vi "Read Decimated Traces.vi"(8 "Error In":errorcluster, 11 "BNT_DSCXtGraph in":refnum<class "BNT_DSCXtGraph.lvclass">) -> (0 "Error Out":errorcluster, 3 "BNT_DSCXtGraph out":refnum<class "BNT_DSCXtGraph.lvclass">)   [LabVIEW 2021, in "BNT_DSCXtGraph.lvlib" / "BNT_DSCXtGraph.lvclass"]
uses:
  BNT_DSCXtGraph.lvclass
  BNT_DSCXtGraph.lvclass/BNT_DSCXtGraph.ctl
  <vilib>/lvdsc/historical/Read Traces (Numeric).vi
  <vilib>/lvdsc/NI_DSC.lvlib
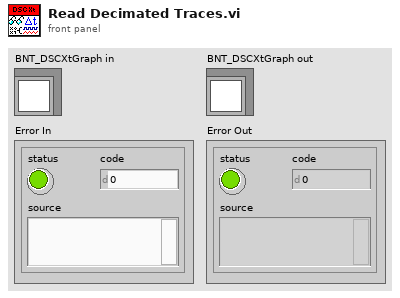
[diagram p1: front panel]
types:
  T1 = cluster{"Start Times":timestamp, "Stop Time":timestamp}
  T2 = cluster{"interpolate data (F)":bool, "extrapolate to now (F)":bool, "remove data breaks (F)":bool, "interpolation interval (1 s)":dbl, "maintain trending info (T)":bool}
  T3 = cluster{"timestamps":timestamp[], "data":dbl[]}[]
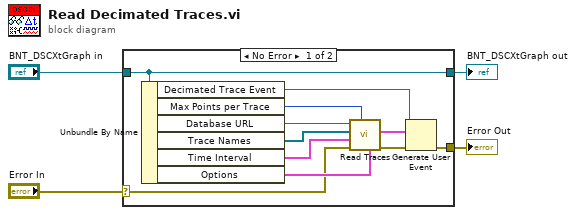
[diagram p0: block diagram]
diagram:
  n1 = case shown="No Error" "Error In" {
    selector: "Error In" -> [w9 w17]
    tunnel: [w6 w17] -> w1
    tunnel: [w15 w16] -> w2
    tunnel: "BNT_DSCXtGraph in" -> [w15 w16]
    frame No Error {
      n2 = Unbundle By Name(w15) -> ("Decimated Trace Event"=w8:refnum<user-event>, "Max Points per Trace"=w11:i32, "Database URL"=w14:path, "Trace Names"=w13:refnum<k21>[], "Time Interval"=w10:T1, "Options"=w12:T2)
      n3 = call-poly <vilib>:"Read Traces.vi"("options"=w12, "max points per trace (all)"=w11, "error in (no error)"=w9, "time interval"=w10, "trace names"=w13, "database URL"=w14) -> ("error out"=w7:errorcluster, "historical traces"=w5:T3)  [unwired: 2 in, 2 out]
      n4 = Generate User Event(user event=w8, event data cluster=w5, error in=w7) -> (error out=w6:errorcluster)  [unwired: 1 in, 1 out]
    }
    frame Error {
    }
  }
  "Error Out" <- w1
  "BNT_DSCXtGraph out" <- w2
